vi "GenerateStimulusOutputs_2P.vi"(0 "Trial duration (min)":dbl, 1 "Rest duration(s)":dbl, 2 "trial offset (s)":dbl, 3 "Left Pad":dbl, 4 "Right Pad":dbl, 5 "Auditory":dbl, 6 "LED":dbl, 8 "LED Stim Duration (s)":dbl, 9 "LED Stim Parameters":cluster{"Fs":dbl, "Samples":dbl}, 10 "LED Frequency":dbl, 11 "Sol Stim Parameters":cluster{"Fs":dbl, "Samples":dbl}, 12 "LED duty cycle (%)":dbl, 14 "Sol Stim Duration (s)":dbl, 16 "Sol Frequency":dbl, 18 "Sol Duty Cycle (%)":dbl) -> (20 "Solenoid Stim Waveforms":digitalwaveform(graph), 22 "Stimulus Digital Outputs":digitalwaveform[](array[waveform]), 24 "Left Pad Out":digitalwaveform(graph), 25 "Auditory Out":digitalwaveform(graph), 26 "Right Pad Out":digitalwaveform(graph), 27 "LED Out":digitalwaveform(graph))   [LabVIEW 2020]
uses:
  <vilib>/Waveform/DWDTOps.llb/DWDT Analog to Digital.vi
  <vilib>/Waveform/DWDTOps.llb/DWDT Digital to Analog.vi
  <vilib>/measure/NI_MABase.lvlib
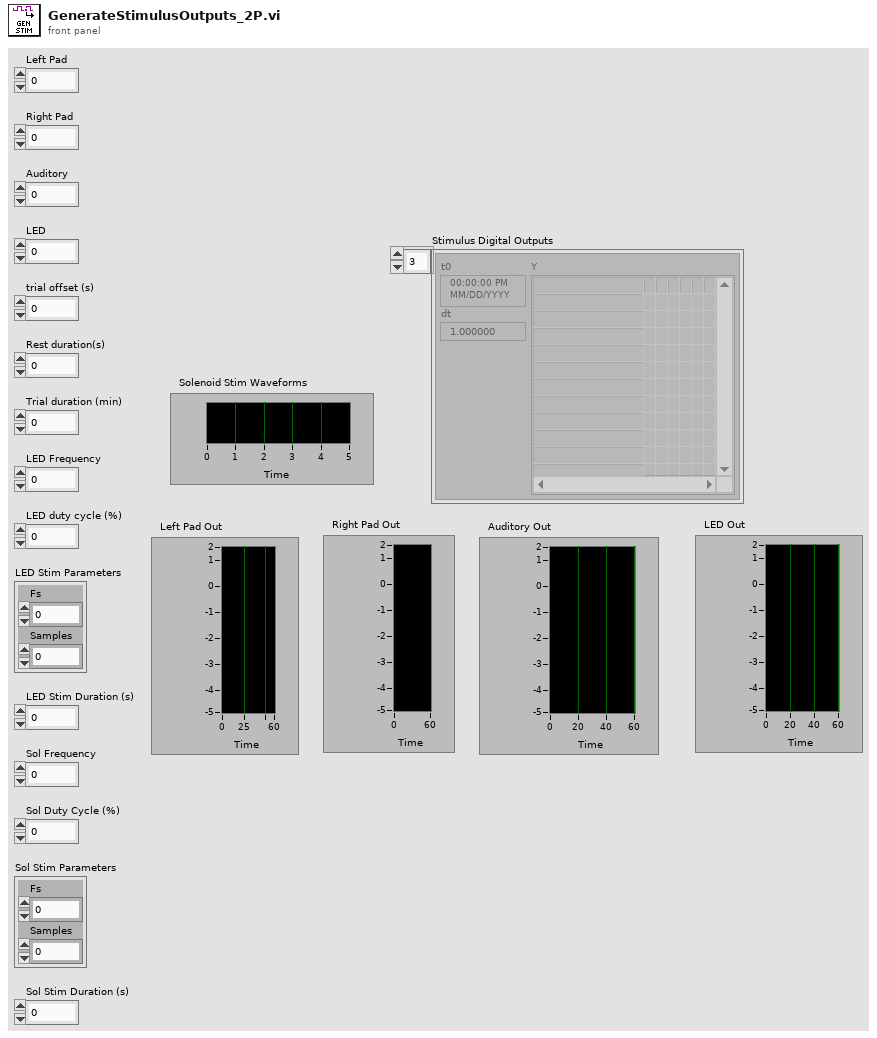
[diagram p1: front panel]
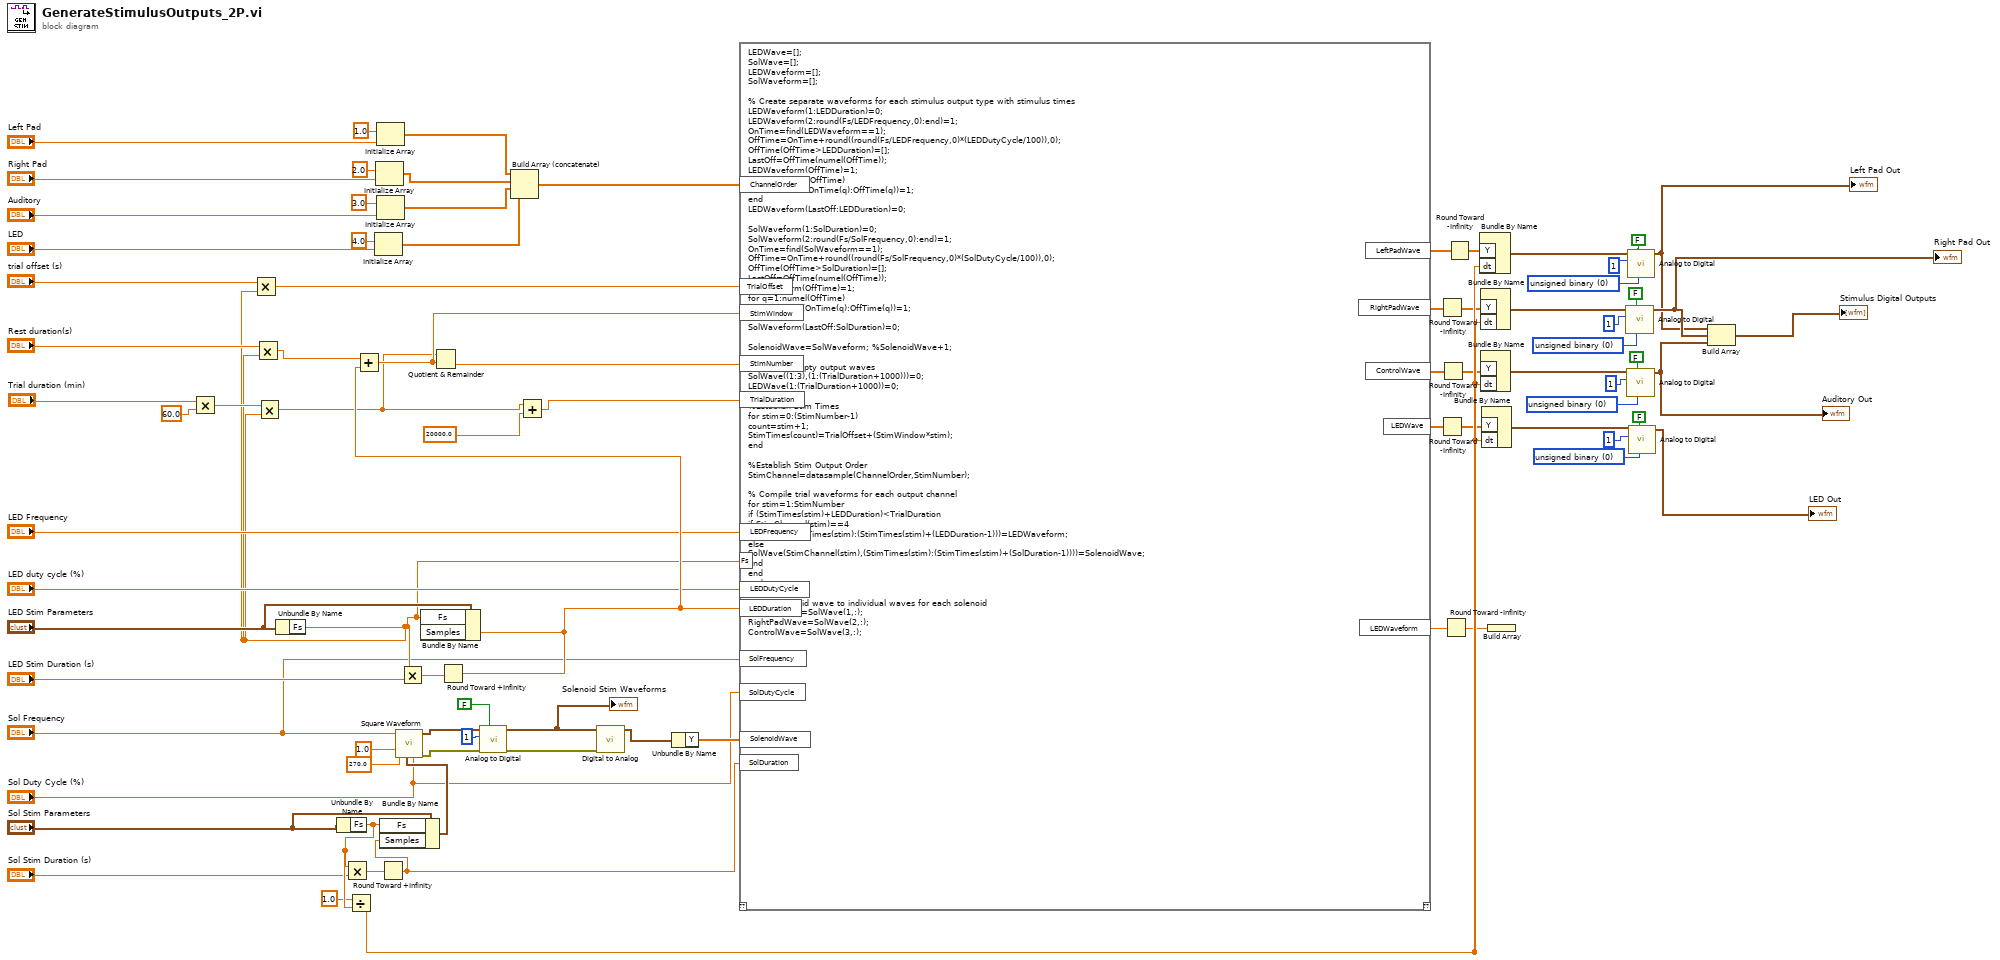
[diagram p0: block diagram]
diagram:
  w80 = u16 0 items=["unsigned binary", "offset binary", "2's complement"] ("data format (offset binary)")
  w79 = u16 0 items=["unsigned binary", "offset binary", "2's complement"] ("data format (offset binary)")
  w78 = u16 0 items=["unsigned binary", "offset binary", "2's complement"] ("data format (offset binary)")
  w77 = u16 0 items=["unsigned binary", "offset binary", "2's complement"] ("data format (offset binary)")
  n1 = Multiply(x="Trial duration (min)", y=60.0) -> (x*y=w23:dbl)
  n2 = Unbundle By Name("LED Stim Parameters") -> ("Fs"=w18:dbl)
  n3 = Multiply(x="trial offset (s)", y=w18) -> (x*y=w68:dbl)
  n4 = Multiply(x="Rest duration(s)", y=w18) -> (x*y=w27:dbl)
  n5 = Multiply(x=w23, y=w18) -> (x*y=w3:dbl)
  n6 = Unbundle By Name("Sol Stim Parameters") -> ("Fs"=w73:dbl)
  n7 = Multiply(x=w73, y="Sol Stim Duration (s)") -> (x*y=w55:dbl)
  n8 = Divide(x=1.0, y=w73) -> (x/y=w17:dbl)
  n9 = Initialize Array(4.0 ("element"), "LED") -> (w39:dbl[])
  n10 = Initialize Array(2.0 ("element"), "Right Pad") -> (w37:dbl[])
  n11 = Initialize Array(1.0 ("element"), "Left Pad") -> (w36:dbl[])
  n12 = Initialize Array(3.0 ("element"), "Auditory") -> (w38:dbl[])
  n13 = Round Toward +Infinity(x=w55) -> (ceil(x): smallest int >= x=w56:dbl)
  n14 = Bundle By Name(cluster="Sol Stim Parameters", "Fs"=w73, "Samples"=w56) -> (w43:cluster{"Fs":dbl, "Samples":dbl})
  n15 = call <vilib>:"Square Waveform.vi"("duty cycle (%)"="Sol Duty Cycle (%)", "sampling info"=w43, "phase"=270.0, "amplitude"=1.0, "frequency"="Sol Frequency") -> ("error out"=w46:errorcluster, "signal out"=w49:waveform(dbl))  [unwired: 5 in]
  n16 = Multiply(x=w18, y="LED Stim Duration (s)") -> (x*y=w54:dbl)
  n17 = Round Toward +Infinity(x=w54) -> (ceil(x): smallest int >= x=w82:dbl)
  n18 = Add(x=w27, y=w82) -> (x+y=w69:dbl)
  n19 = Bundle By Name(cluster="LED Stim Parameters", "Fs"=w18, "Samples"=w82) -> ()  [unwired: 1 out]
  n20 = Quotient & Remainder(x=w3, y=w69) -> (floor(x/y)=w66:dbl)  [unwired: 1 out]
  n21 = call-poly <vilib>:"Analog to Digital.vi"("compress digital (T)"=FALSE, "error in (no error)"=w46, "resolution (16 bit)"=1, "analog waveform"=w49) -> ("error out"=w47:errorcluster, "digital waveform"=w71:digitalwaveform)  [unwired: 4 in, 2 out]
  "Solenoid Stim Waveforms" <- w71
  n22 = Build Array (concatenate)(w36, w37, w38, w39) -> (w67:dbl[])
  n23 = Add(x=w3, y=20000.0) -> (x+y=w1:dbl)
  n24 = call-poly <vilib>:"Digital to Analog.vi"("error in (no error)"=w47, "digital waveform"=w71) -> ("analog waveform"=w45:waveform(dbl))  [unwired: 6 in, 3 out]
  n25 = Unbundle By Name(w45) -> ("Y"=w65:dbl[])
  n26 = script code="LEDWave=[];\nSolWave=[];\nLEDWaveform=[];\nSolWaveform=[];\n\n% Create separate waveforms for each stimulus output type with stimulus times\nLEDWaveform(1:LEDDuration)=0;\nLEDWaveform(2:round(Fs/LEDFrequency,0):end)=1;\nOnTime=find(LEDWaveform==1);\nOffTime=OnTime+round((round(Fs/LEDFrequency,0)*(LEDDutyCycle/100)),0);\nOffTime(OffTime>LEDDuration)=[];\nLastOff=OffTime(numel(OffTime));\nLEDWaveform(OffTime)=1;\nfor q=1:numel(OffTime)\nLEDWaveform(OnTime(q):OffTime(q))=1;\nend\nLEDWaveform(LastOff:LEDDuration)=0;\n\nSolWaveform(1:SolDuration)=0;\nSolWaveform(2:round(Fs/SolFrequency,0):end)=1;\nOnTime=find(SolWaveform==1);\nOffTime=OnTime+round((round(Fs/SolFrequency,0)*(SolDutyCycle/100)),0);\nOffTime(OffTime>SolDuration)=[];\nLastOff=OffTime(numel(OffTime));\nSolWaveform(OffTime)=1;\nfor q=1:numel(OffTime)\nSolWaveform(OnTime(q):OffTime(q))=1;\nend\nSolWaveform(LastOff:SolDuration)=0;\n\nSolenoidWave=SolWaveform; %SolenoidWave+1;\n\n%initialize empty output waves\nSolWave((1:3),(1:(TrialDuration+1000)))=0;\nLEDWave(1:(TrialDuration+1000))=0;\n\n%Establish Stim Times\nfor stim=0:(StimNumber-1)\ncount=stim+1;\nStimTimes(count)=TrialOffset+(StimWindow*stim);\nend\n\n%Establish Stim Output Order\nStimChannel=datasample(ChannelOrder,StimNumber); \n\n% Compile trial waveforms for each output channel\nfor stim=1:StimNumber\nif (StimTimes(stim)+LEDDuration)<TrialDuration\nif StimChannel(stim)==4\nLEDWave(StimTimes(stim):(StimTimes(stim)+(LEDDuration-1)))=LEDWaveform;\nelse \nSolWave(StimChannel(stim),(StimTimes(stim):(StimTimes(stim)+(SolDuration-1))))=SolenoidWave;\nend\nend\nend\n\n%Split solenoid wave to individual waves for each solenoid\nLeftPadWave=SolWave(1,:);\nRightPadWave=SolWave(2,:);\nControlWave=SolWave(3,:);"("StimNumber"=w66, "ChannelOrder"=w67, "TrialDuration"=w1, "SolenoidWave"=w65, "LEDDuration"=w82, "SolDuration"=w56, "TrialOffset"=w68, "StimWindow"=w69, "LEDDutyCycle"="LED duty cycle (%)", "LEDFrequency"="LED Frequency", "Fs"=w18, "SolFrequency"="Sol Frequency", "SolDutyCycle"="Sol Duty Cycle (%)") -> ("LeftPadWave"=w83:dbl[], "RightPadWave"=w63:dbl[], "ControlWave"=w64:dbl[], "LEDWave"=w74:dbl[], "LEDWaveform"=w14:dbl)  [unwired: 1 in, 1 out]
  n27 = Round Toward -Infinity(1:w63) -> (0:w12:dbl[])
  n28 = Round Toward -Infinity(1:w74) -> (0:w15:dbl[])
  n29 = Round Toward -Infinity(1:w64) -> (0:w10:dbl[])
  n30 = Round Toward -Infinity(1:w14) -> (0:w13:dbl)
  n31 = Round Toward -Infinity(1:w83) -> (0:w11:dbl[])
  n32 = Bundle By Name("Y"=w11, "dt"=w17) -> (w16:waveform(dbl))  [unwired: 1 in]
  n33 = Bundle By Name("Y"=w12, "dt"=w17) -> (w81:waveform(dbl))  [unwired: 1 in]
  n34 = Bundle By Name("Y"=w10, "dt"=w17) -> (w76:waveform(dbl))  [unwired: 1 in]
  n35 = Bundle By Name("Y"=w15, "dt"=w17) -> (w75:waveform(dbl))  [unwired: 1 in]
  n36 = Build Array(w13) -> ()  [unwired: 1 out]
  n37 = call-poly <vilib>:"Analog to Digital.vi"("data format (offset binary)"=w78, "compress digital (T)"=FALSE, "resolution (16 bit)"=1, "analog waveform"=w81) -> ("digital waveform"=w5:digitalwaveform)  [unwired: 4 in, 3 out]
  "Right Pad Out" <- w5
  n38 = call-poly <vilib>:"Analog to Digital.vi"("data format (offset binary)"=w79, "compress digital (T)"=FALSE, "resolution (16 bit)"=1, "analog waveform"=w76) -> ("digital waveform"=w6:digitalwaveform)  [unwired: 4 in, 3 out]
  "Auditory Out" <- w6
  n39 = call-poly <vilib>:"Analog to Digital.vi"("data format (offset binary)"=w77, "compress digital (T)"=FALSE, "resolution (16 bit)"=1, "analog waveform"=w16) -> ("digital waveform"=w4:digitalwaveform)  [unwired: 4 in, 3 out]
  "Left Pad Out" <- w4
  n40 = call-poly <vilib>:"Analog to Digital.vi"("data format (offset binary)"=w80, "compress digital (T)"=FALSE, "resolution (16 bit)"=1, "analog waveform"=w75) -> ("digital waveform"=→"LED Out":digitalwaveform)  [unwired: 4 in, 3 out]
  n41 = Build Array(w4, w5, w6) -> (→"Stimulus Digital Outputs":digitalwaveform[])
